vi "Conditionning - Time Windowing (using TVM).vi"(0 "reference in":refnum<class "GSwFormDSP.lvclass">, 5 "error in (no error)":errorcluster, 7 "Ref Ch. Index":i32) -> (14 "reference in":refnum<class "GSwFormDSP.lvclass">, 19 "error out":errorcluster)   [LabVIEW 2020, in "GSwFormDSP.lvclass"]
uses:
  GSwFormDSP.lvclass
  Generic Utilities_class/Generic Utilities.lvclass
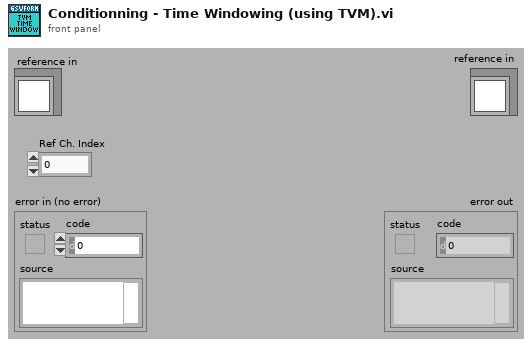
[diagram p1: front panel]
types:
  T1 = enum16{"RMS", "Absolute Peak", "Range", "Standard Deviation", "Variance", "Skewness", "Kurtosis"}
  T2 = typedef "GSwFormDSP.lvclass/ObjectAttributesRef.ctl" = refnum<data-value>
  T3 = typedef "GSwFormDSP.lvclass/ObjectAttributes.ctl" = cluster{"Wform Ref":refnum<data-value>, "Nb Signals":i32, "Spectral Function Parameters":T4, "FFT":waveform(cdb)[], "Nb FFT":i32, "Nb Averages":i32[], "Reference Indexes":i32[], "Response Indexes":i32[], "Coherence":waveform(dbl)[], "TDF Parameters":T6, "DAQ":cluster{"Duration (sec)":dbl, "Buffer Size (Samples)":i32, "Offset (Samples)":i32}, "Filter Impulse Response (TDF)":waveform(dbl), "Sound Playback":T7}
  T4 = typedef "GSwFormDSP.lvclass/Spectral Parameters.ctl" = cluster{"Frequency resolution (Hz)":dbl, "Overlap":dbl, "Window":T5}
  T5 = typedef "NI_AALPro.lvlib/windowTd.ctl" = u32
  T6 = typedef "GSwFormDSP.lvclass/TDF Parameters.ctl" = cluster{"Filter":enum32{"Lowpass", "Highpass", "Bandpass", "Bandstop"}, "Type:":enum16{"Butterworth", "Chebyshev", "Inv Chebyshev", "Elliptic", "Bessel"}, "LP cutoff freq":dbl, "HP cutoff freq":dbl, "Order":i32, "passband ripple (dB)":dbl, "stopband attenuation (dB)":dbl, "Phaseless Filter":bool, "Include Fade IN and OUT":bool}
  T7 = typedef "GSwFormDSP.lvclass/Sound Playback.ctl" = cluster{"Timer start (ms)":u32, "task ID":T8, "Cursor Init Location (s)":dbl, "SC Volume":dbl}
  T8 = typedef "Sound Output Task ID.ctl" = u32
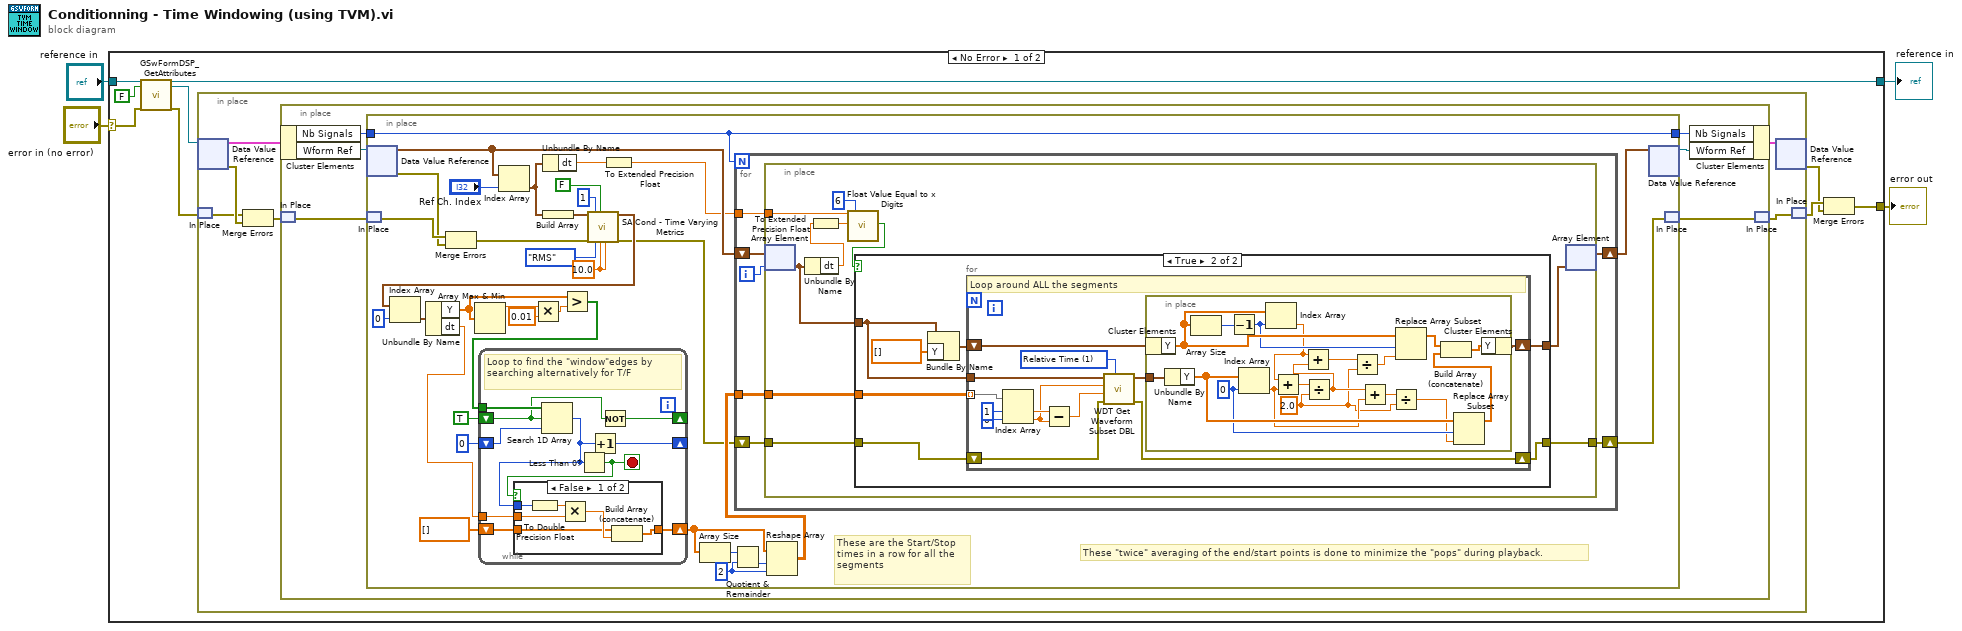
[diagram p0: block diagram]
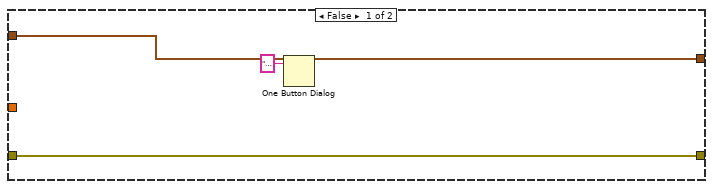
[diagram p3: hidden frame]
diagram:
  n1 = case shown="No Error" "error in (no error)" {
    selector: "error in (no error)" -> [w10 w136]
    tunnel: [w13 w136] -> w3
    tunnel: [w8 w135] -> w1
    tunnel: "reference in" -> [w11 w135]
    frame No Error {
      n2 = call "GSwFormDSP_GetAttributes.vi"("reference in"=w11, "return data? (T)"=FALSE, "error in (no error)"=w10) -> ("reference out"=w8:refnum<class "GSwFormDSP.lvclass">, "attributes ref"=w9:T2, "error out"=w7:errorcluster)  [unwired: 13 in, 1 out]
      n3 = in-place {
        n4 = in-place-dvr #1(w9) -> (w17:T3, w19:errorcluster)
        n5 = in-place-match #2(w7) -> (w18:errorcluster)
        n6 = Merge Errors(w18, w19) -> (w16:errorcluster)
        n7 = in-place {
          n8 = in-place-cluster #3(w17) -> ("Nb Signals"=w21:i32, "Wform Ref"=w25:refnum<data-value>)
          n9 = in-place-match #4(w16) -> (w23:errorcluster)
          n10 = in-place {
            in-place-border: w21 -> [w45]
            in-place-border: [w45] -> w20
            w36 = 2 ("dimension size")
            w54 = 10.0 ("Step (ms)")
            # "These \"twice\" averaging of the end/start points is done to minimize the \"pops\" during playback."
            # "These are the Start/Stop times in a row for all the segments"
            n11 = in-place-dvr #5(w25) -> (w44:waveform(dbl)[], w58:errorcluster)
            n12 = in-place-match #6(w23) -> (w59:errorcluster)
            n13 = Merge Errors(w59, w58) -> (w57:errorcluster)
            n14 = Index Array(array=w44, index="Ref Ch. Index") -> (element=w40:waveform(dbl))
            n15 = Unbundle By Name(w40) -> ("dt"=w30:dbl)
            n16 = Build Array(w40) -> (w52:waveform(dbl)[])
            n17 = call "SA Cond - Time Varying Metrics.vi"("wForm IN"=w52, "error in (no error)"=w57, "Nb Signals"=1, "Trend Type"=T1."RMS", "Anotate Signal Name"=FALSE, "Step (ms)"=w54, "Length (ms)"=w54) -> ("wForm OUT"=w50:waveform(dbl)[], "error out"=w28:errorcluster)  [unwired: 11 in]
            n18 = Index Array(array=w50, index=0) -> (element=w39:waveform(dbl))
            n19 = Unbundle By Name(w39) -> ("Y"=w41:dbl[], "dt"=w26:dbl)
            n20 = Array Max & Min(array=w41) -> (max value=w49:dbl)  [unwired: 3 out]
            n21 = Multiply(x=w49, y=0.01) -> (x*y=w47:dbl)
            n22 = Greater?(x=w41, y=w47) -> (0:w31:bool[])
            n23 = while {
              tunnel: w31 -> [w69]
              shift-right: [w67] -> _
              shift-left: 0 -> [w68]
              shift-right: [w66] -> _
              shift-left: TRUE -> [w65]
              tunnel: w26 -> [w62]
              shift-right: [w60] -> w38
              shift-left: dbl[] [] -> [w61]
              stop <- w64 stop-if-true
              # "Loop to find the \"window\"edges by searching alternatively for T/F"
              n24 = Search 1D Array(1D array=w69, element=w65, start index (0)=w68) -> (index of element=w63:i32)
              n25 = Less Than 0?(x=w63) -> (x < 0?=w64:bool)
              n26 = case shown="False" w64 {
                tunnel: w63 -> [w74 _]
                tunnel: w62 -> [w73 _]
                tunnel: w61 -> [w71 w76]
                tunnel: [w70 w76] -> w60
                frame False {
                  n27 = To Double Precision Float(number=w74) -> (double precision float=w75:dbl)
                  n28 = Multiply(x=w75, y=w73) -> (x*y=w72:dbl)
                  n29 = Build Array (concatenate)(w71, w72) -> (w70:dbl[])
                }
                frame True {
                }
              }
              n30 = Increment(x=w63) -> (x+1=w67:i32)
              n31 = Not(x=w65) -> (.not. x?=w66:bool)
            }
            n32 = To Extended Precision Float(1:w30) -> (0:w42:ext)
            n33 = Array Size(array=w38) -> (size(s)=w35:i32)
            n34 = Quotient & Remainder(x=w35, y=w36) -> (floor(x/y)=w37:i32)  [unwired: 1 out]
            n35 = Reshape Array(w38, w37, w36) -> (w29:dbl[][])
            n36 = for {
              N: w45 -> [_]
              shift-right: [w81] -> w43
              shift-left: w44 -> [w83]
              tunnel: w42 -> [w80]
              tunnel: w29 -> [w79]
              shift-right: [w77] -> w27
              shift-left: w28 -> [w78]
              i -> [w82]
              n37 = in-place {
                in-place-border: w80 -> [w93]
                in-place-border: w79 -> [w87]
                in-place-border: w78 -> [w85]
                in-place-border: [w84] -> w77
                n38 = in-place-array #7(w83, w82) -> (w89:waveform(dbl))
                n39 = Unbundle By Name(w89) -> ("dt"=w91:dbl)
                n40 = To Extended Precision Float(1:w91) -> (0:w92:ext)
                n41 = call "Float Value Equal to x Digits.vi"("Value A"=w93, "Value B"=w92, "Desired Number of matching digits"=6) -> ("Equal?"=w88:bool)  [unwired: 16 in]
                n42 = case shown="True" w88 {
                  tunnel: [w95 w103] -> w86
                  tunnel: w89 -> [w95 w99]
                  tunnel: w87 -> [_ w102]
                  tunnel: w85 -> [w94 w98]
                  tunnel: [w94 w97] -> w84
                  frame False {
                    n43 = One Button Dialog(message="Warning, the silence part of a signal could NOT be removed because the sampling rate OR the number of samples does NOT match the reference signal sampling rate OR number of samples.") -> ()  [unwired: 1 in, 1 out]
                  }
                  frame True {
                    n44 = Bundle By Name(cluster=w99, "Y"=dbl[] []) -> (w100:waveform(dbl))
                    n45 = for {
                      shift-right: [w106] -> w103
                      shift-left: w100 -> [w107]
                      tunnel: w102 -> [w111] mode=indexing
                      tunnel: w99 -> [w115]
                      shift-right: [w104] -> w97
                      shift-left: w98 -> [w105]
                      w116 = u16 1 items=["Samples", "Relative Time"] ("start/duration format")
                      # "Loop around ALL the segments"
                      n46 = Index Array(array=w111, index #1=1 ("index"), index #2=0 ("index")) -> (element #1=w112:dbl, element #2=w109:dbl)
                      n47 = Subtract(x=w112, y=w109) -> (x-y=w110:dbl)
                      n48 = call <vilib>:"WDT Get Waveform Subset DBL.vi"("start/duration format"=w116, "error in (no error)"=w105, "duration"=w110, "start samples/time"=w109, "waveform in"=w115) -> ("error out"=w104:errorcluster, "waveform out"=w108:waveform(dbl))  [unwired: 1 in, 2 out]
                      n49 = in-place {
                        in-place-border: w108 -> [w134]
                        w118 = 2.0 ("y")
                        w130 = 0 ("index")
                        n50 = in-place-cluster #8(w107) -> ("Y"=w129:dbl[])
                        n51 = Unbundle By Name(w134) -> ("Y"=w131:dbl[])
                        n52 = Array Size(array=w129) -> (size(s)=w133:i32)
                        n53 = Decrement(x=w133) -> (x-1=w127:i32)
                        n54 = Index Array(array=w131, index=w130) -> (element=w120:dbl)
                        n55 = Index Array(array=w129, index=w127) -> (element=w124:dbl)
                        n56 = Add(x=w124, y=w120) -> (x+y=w125:dbl)
                        n57 = Divide(x=w125, y=w118) -> (x/y=w121:dbl)
                        n58 = Add(x=w124, y=w121) -> (x+y=w123:dbl)
                        n59 = Divide(x=w123, y=w118) -> (x/y=w122:dbl)
                        n60 = Add(x=w121, y=w120) -> (x+y=w119:dbl)
                        n61 = Divide(x=w119, y=w118) -> (x/y=w117:dbl)
                        n62 = Replace Array Subset(array=w129, new element=w122, index=w127) -> (w128:dbl[])
                        n63 = Replace Array Subset(array=w131, new element=w117, index=w130) -> (w126:dbl[])
                        n64 = Build Array (concatenate)(w128, w126) -> (w132:dbl[])
                        n65 = in-place-cluster #8("Y"=w132) -> (w106:waveform(dbl))
                      }
                    }
                  }
                }
                n66 = in-place-array #7(w86) -> (w81:waveform(dbl)[])  [unwired: 1 out]
              }
            }
            n67 = in-place-dvr #5(w43) -> (w24:refnum<data-value>)  [unwired: 1 out]
            n68 = in-place-match #6(w27) -> (w22:errorcluster)
          }
          n69 = in-place-cluster #3("Nb Signals"=w20, "Wform Ref"=w24) -> (w15:T3)
          n70 = in-place-match #4(w22) -> (w14:errorcluster)
        }
        n71 = in-place-dvr #1(w15) -> (w5:errorcluster)  [unwired: 1 out]
        n72 = in-place-match #2(w14) -> (w6:errorcluster)
      }
      n73 = Merge Errors(w6, w5) -> (w13:errorcluster)
    }
    frame Error {
    }
  }
  "error out" <- w3
  "reference in" <- w1
